vi "generate_trajectory.vi"(0 "TrajectoryTS090820Circular2D in":refnum<class "TrajectoryTS090820Circular2D.lvclass">, 1 "trajectory params":T1, 5 "error in (no error)":errorcluster) -> (14 "TrajectoryTS090820Circular2D out":refnum<class "TrajectoryTS090820Circular2D.lvclass">, 15 "trajectory":cluster{dbl[], dbl[], dbl[], dbl[]}, 19 "error out":errorcluster)   [LabVIEW 2010, in "TrajectoryTS090820Circular2D.lvclass"]
uses:
  TrajectoryTS090820Circular2D.lvclass
  TrajectoryTS090820Circular2D.lvclass/TrajectoryTS090820Circular2D.ctl
panel:
  out "dump factor":dbl=1.1
  out "Spiral?":bool
  out "points BEFORE equal-distribution":cluster{dbl, dbl}[](graph)
  out "intensity":dbl[](array[numeric])
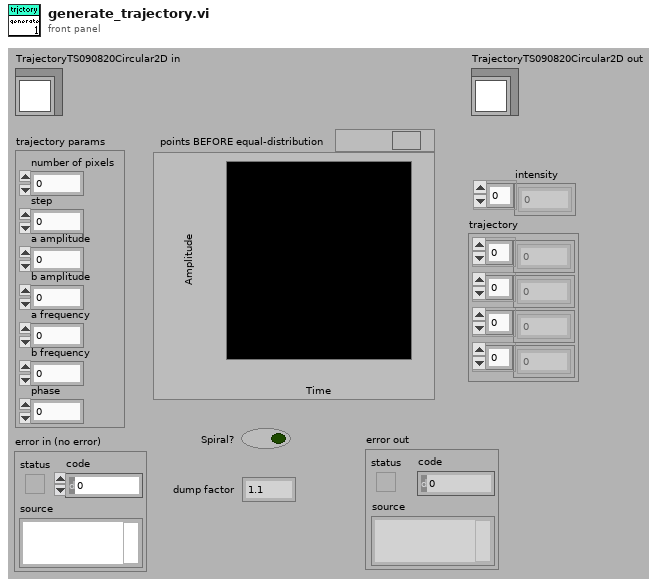
[diagram p1: front panel]
types:
  T1 = cluster{"number of pixels":i32, "step":dbl, "a amplitude":dbl, "b amplitude":dbl, "a frequency":dbl, "b frequency":dbl, "phase":dbl}
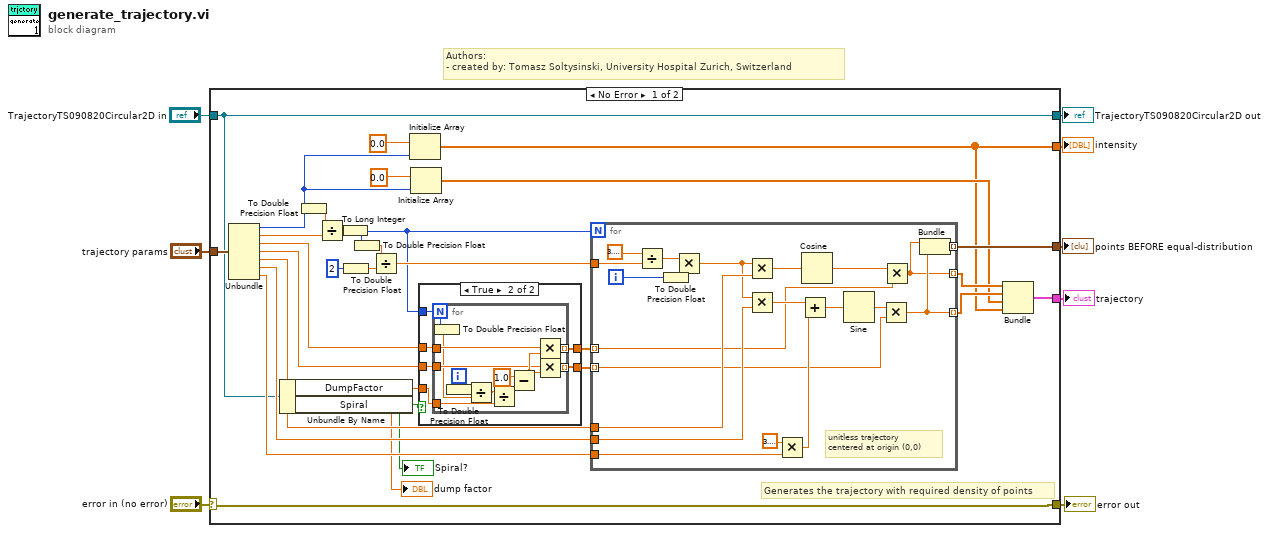
[diagram p0: block diagram]
diagram:
  # "Authors: \n- created by: Tomasz Soltysinski, University Hospital Zurich, Switzerland"
  n1 = case shown="No Error" "error in (no error)" {
    selector: "error in (no error)" -> [w37 w86]
    tunnel: [w37 w86] -> w8
    tunnel: [w11 w85] -> w6
    tunnel: "TrajectoryTS090820Circular2D in" -> [w11 w85]
    tunnel: [w18 _] -> w5
    tunnel: "trajectory params" -> [w28 _]
    tunnel: [w22 _] -> w3
    tunnel: [w17 _] -> w2
    frame No Error {
      # "Generates the trajectory with required density of points"
      n2 = Unbundle(w28) -> ("number of pixels"=w27:i32, "step"=w26:dbl, "a amplitude"=w16:dbl, "b amplitude"=w15:dbl, "a frequency"=w25:dbl, "b frequency"=w24:dbl, "phase"=w23:dbl)
      n3 = Unbundle By Name(w11) -> ("DumpFactor"=w9:dbl, "Spiral"=w10:bool)
      "Spiral?" <- w10
      "dump factor" <- w9
      n4 = To Double Precision Float(number=w27) -> (double precision float=w30:dbl)
      n5 = Divide(x=w30, y=w26) -> (x/y=w29:dbl)
      n6 = To Long Integer(number=w29) -> (32bit integer=w12:i32)
      n7 = To Double Precision Float(number=2) -> (double precision float=w36:dbl)
      n8 = To Double Precision Float(number=w12) -> (double precision float=w34:dbl)
      n9 = Divide(x=w34, y=w36) -> (x/y=w31:dbl)
      n10 = Initialize Array(0.0 ("dimension size"), w27) -> (w18:dbl[])
      n11 = Initialize Array(0.0 ("dimension size"), w27) -> (w19:dbl[])
      n12 = case shown="True" w10 {
        tunnel: w16 -> [w42 w50]
        tunnel: w15 -> [w41 w48]
        tunnel: [w39 w47] -> w13
        tunnel: [w40 w49] -> w14
        tunnel: w12 -> [w38 w46]
        tunnel: w9 -> [_ w45]
        frame False {
          n13 = for {
            N: w38 -> [_]
            tunnel: w42 -> [w44]
            tunnel: w41 -> [w43]
            tunnel: [w44] -> w40 mode=indexing
            tunnel: [w43] -> w39 mode=indexing
          }
        }
        frame True {
          n14 = for {
            N: w46 -> [w59]
            tunnel: w50 -> [w63]
            tunnel: [w62] -> w49 mode=indexing
            tunnel: w48 -> [w56]
            tunnel: [w61] -> w47 mode=indexing
            tunnel: w45 -> [w60]
            i -> [w53]
            n15 = To Double Precision Float(number=w59) -> (double precision float=w51:dbl)
            n16 = To Double Precision Float(number=w53) -> (double precision float=w52:dbl)
            n17 = Divide(x=w52, y=w51) -> (x/y=w55:dbl)
            n18 = Divide(x=w55, y=w60) -> (x/y=w54:dbl)
            n19 = Subtract(x=1.0, y=w54) -> (x-y=w57:dbl)
            n20 = Multiply(x=w63, y=w57) -> (x*y=w62:dbl)
            n21 = Multiply(x=w56, y=w57) -> (x*y=w61:dbl)
          }
        }
      }
      n22 = for {
        N: w12 -> [_]
        tunnel: w23 -> [w78]
        tunnel: w31 -> [w81]
        tunnel: w25 -> [w77]
        tunnel: w24 -> [w76]
        tunnel: [w71] -> w21 mode=indexing
        tunnel: [w72] -> w20 mode=indexing
        tunnel: [w70] -> w22 mode=indexing
        tunnel: w14 -> [w65] mode=indexing
        tunnel: w13 -> [w64] mode=indexing
        i -> [w66]
        # "unitless trajectory\ncentered at origin (0,0)"
        n23 = Divide(x=3.141592653589793, y=w81) -> (x/y=w84:dbl)
        n24 = To Double Precision Float(number=w66) -> (double precision float=w74:dbl)
        n25 = Multiply(x=w84, y=w74) -> (x*y=w69:dbl)
        n26 = Multiply(x=w69, y=w77) -> (x*y=w68:dbl)
        n27 = Multiply(x=w69, y=w76) -> (x*y=w75:dbl)
        n28 = Multiply(x=3.141592653589793, y=w78) -> (x*y=w80:dbl)
        n29 = Add(x=w75, y=w80) -> (x+y=w67:dbl)
        n30 = Cosine(x=w68) -> (cos(x)=w73:dbl)
        n31 = Sine(x=w67) -> (sin(x)=w82:dbl)
        n32 = Multiply(x=w82, y=w64) -> (x*y=w72:dbl)
        n33 = Multiply(x=w73, y=w65) -> (x*y=w71:dbl)
        n34 = Bundle(w71, w72) -> (w70:cluster{dbl, dbl})  [unwired: 1 in]
      }
      n35 = Bundle(w21, w20, w19, w18) -> (w17:cluster{dbl[], dbl[], dbl[], dbl[]})  [unwired: 1 in]
    }
    frame Error {
    }
  }
  "error out" <- w8
  "TrajectoryTS090820Circular2D out" <- w6
  "intensity" <- w5
  "points BEFORE equal-distribution" <- w3
  "trajectory" <- w2
